vi "MGCC_Commun_PollIndex.vi"(11 "Analog Input Indexes":u16[](array[numeric])) -> (3 "Poll":T1[](array[typedef]))   [LabVIEW 2016]
uses:
  <vilib>/DNP3/DNP3_Master/Start Stop.ctl
  <vilib>/DNP3/DNP3_Master.lvlib
panel:
  out "stop":i32
  out "Numeric":i32
  out "start":u16
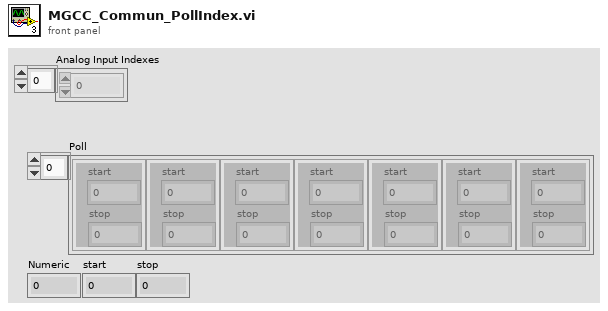
[diagram p1: front panel]
types:
  T1 = typedef "DNP3_Master.lvlib/Start Stop.ctl" = cluster{"start":u16, "stop":u16}
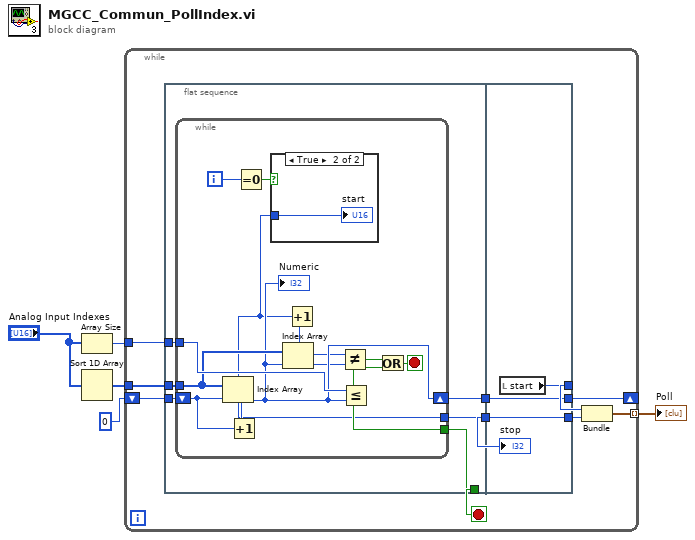
[diagram p0: block diagram]
diagram:
  n1 = Array Size(array="Analog Input Indexes") -> (size(s)=w3:i32)
  n2 = Sort 1D Array(array="Analog Input Indexes") -> (sorted array=w2:u16[])
  n3 = while {
    tunnel: w2 -> [w14]
    tunnel: w3 -> [w15]
    shift-right: [w13] -> _
    shift-left: 0 -> [w12]
    tunnel: [w11] -> w5 mode=indexing
    stop <- w8 stop-if-true
    n4 = flat-sequence {
      tunnel: w15 -> [w21]
      tunnel: w14 -> [w20]
      tunnel: w12 -> [w18]
      tunnel: [w19] -> w10
      tunnel: [w17] -> w8
      tunnel: [w16] -> w7
      tunnel: [w37] -> w13
      tunnel: w10 -> [w37]
      tunnel: [w36] -> w9
      tunnel: w7 -> [w35]
      tunnel: [w35] -> w6
      frame #0 {
        n5 = while {
          tunnel: w21 -> [w33]
          tunnel: w20 -> [w26]
          shift-right: [w25] -> w19
          shift-left: w18 -> [w32]
          tunnel: [w27] -> w17
          tunnel: [w22] -> w16
          i -> [w29]
          stop <- w31 stop-if-true
          n6 = Index Array(array=w26, index=w32) -> (element=w22:u16)
          n7 = Increment(x=w32) -> (x+1=w25:i32)
          "Numeric" <- w25
          n8 = Equal To 0?(x=w29) -> (x = 0?=w28:bool)
          n9 = case shown="True" w28 {
            tunnel: w22 -> [_ w34]
            frame False {
            }
            frame True {
              "start" <- w34
            }
          }
          n10 = Index Array(array=w26, index=w25) -> (element=w23:u16)
          n11 = Increment(x=w22) -> (x+1=w24:u16)
          n12 = Not Equal?(x=w24, y=w23) -> (x != y?=w30:bool)
          n13 = Less Or Equal?(x=w33, y=w25) -> (x <= y?=w27:bool)
          n14 = Or(x=w30, y=w27) -> (x .or. y?=w31:bool)
        }
      }
      frame #1 {
        n15 = local read "start"() -> (w36:u16)
        "stop" <- w35
      }
    }
    n16 = Bundle("start"=w9, w6) -> (w11:cluster{"start":u16, u16})  [unwired: 1 in]
  }
  "Poll" <- w5
